vi "Node ID FGV.vi"(8 "Initialize":T1, 10 "Node Path":path, 11 "Node ID":string) -> (1 "found?":bool, 2 "Node ID":string, 3 "value":map{path, string}(c390))   [LabVIEW 2020, in "SimpleDependencyInspector.lvlib"]
uses:
  SimpleDependencyInspector.lvlib
  FGV Functions--enum.ctl
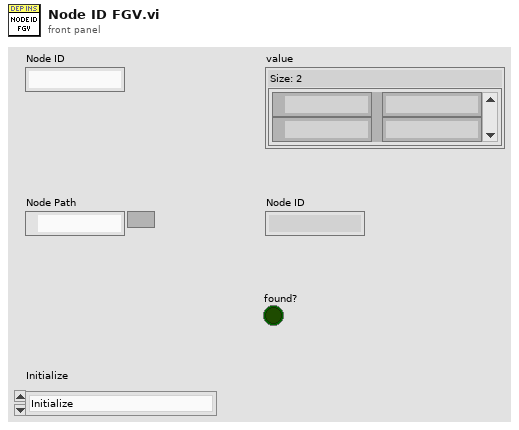
[diagram p1: front panel]
types:
  T1 = typedef "SimpleDependencyInspector.lvlib/FGV Functions--enum.ctl" = enum16{"Initialize", "Get Node ID", "Set Node ID"}
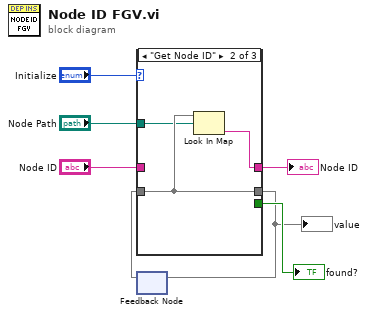
[diagram p0: block diagram]
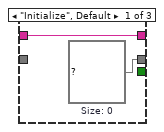
[diagram p2: hidden frame]
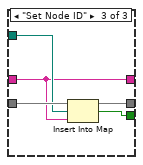
[diagram p3: hidden frame]
diagram:
  n1 = feedback #1() -> (w6:map{path, string})  [unwired: 1 in]
  n2 = case shown="\"Get Node ID\"" "Initialize" {
    tunnel: "Node ID" -> [w8 _ w13]
    tunnel: [w9 w12 w16] -> w2
    tunnel: w6 -> [_ w12 w17]
    tunnel: [_ _ w15] -> w4
    tunnel: "Node Path" -> [_ w11 w14]
    tunnel: [w8 w10 w13] -> w1
    frame "Initialize", Default {
      w9 = map{path, string} {}  # Size: 0
    }
    frame "Get Node ID" {
      n3 = Look In Map(map=w12, key=w11) -> (value=w10:string)  [unwired: 1 in, 1 out]
    }
    frame "Set Node ID" {
      n4 = Insert Into Map(map in=w17, key=w14, value=w13) -> (map out=w16:map{path, string}, key already included?=w15:bool)  [unwired: 1 out]
    }
  }
  "found?" <- w4
  "Node ID" <- w1
  "value" <- w2
  n5 = feedback-in #1(w2) -> ()
